vi "Destroy.vi"(0 "reference in":refnum<class "Test Controller.lvclass">, 5 "error in (no error)":errorcluster) -> (14 "reference out":refnum<class "Test Controller.lvclass">, 19 "error out":errorcluster)   [LabVIEW 2016, in "Test Controller.lvclass"]
doc: "Destructor."
uses:
  Test Controller.lvclass
  <vilib>/addons/_AddQ/G#Object/G#Object.lvclass
  C:/Program Files (x86)/National Instruments/LabVIEW 2016/vi.lib/addons/_AddQ/G#Object/G#Object.lvclass
  APP/python_class/python.lvclass
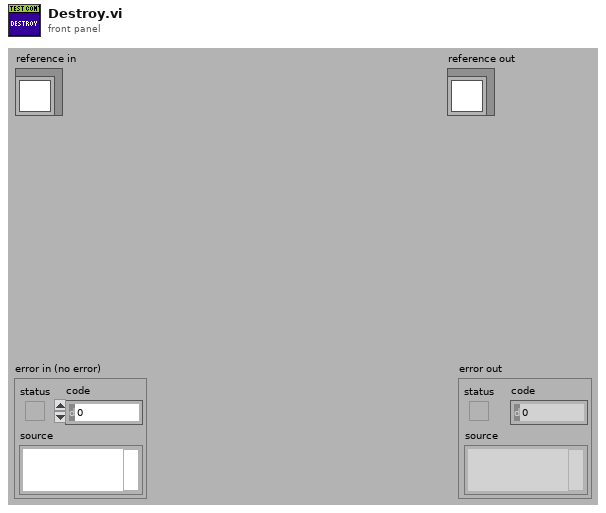
[diagram p1: front panel]
types:
  T1 = typedef "Test Controller.lvclass/ObjectAttributes.ctl" = cluster{"MyAttribute":dbl, "Devices Controller_ref":refnum<class "Devices Controller.lvclass">, "File Controller_ref":refnum<class "File Controller.lvclass">, "Items Controller_ref":refnum<class "Items Controller.lvclass">, "GUI Controller_ref":refnum<class "GUI Controller.lvclass">, "NotificationController_ref":refnum<class "Notification Controller.lvclass">, "PartsTracking Controller_ref":refnum<class "PartsTracking Controller.lvclass">}
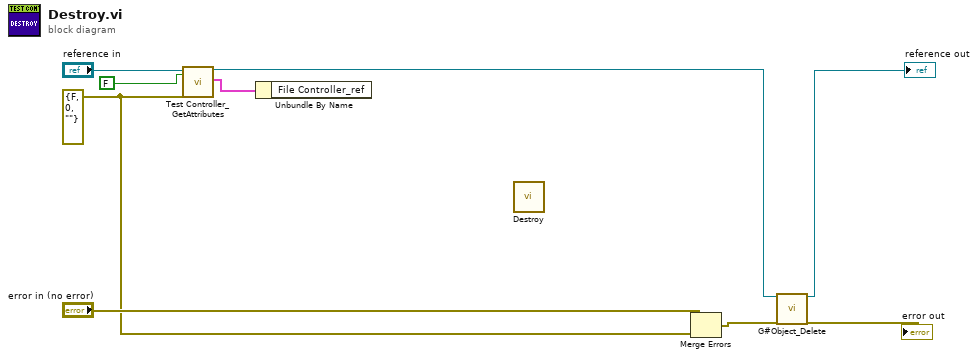
[diagram p0: block diagram]
diagram:
  w10 = errorcluster {"status"=FALSE, "code"=0, "source"=""} ("error in (no error)")
  n1 = call "Test Controller_GetAttributes.vi"("reference in"="reference in", "return data? (T)"=FALSE ("simple info"), "error in (no error)"=w10) -> ("reference out"=w7:refnum<class "Test Controller.lvclass">, "attributes"=w4:T1, "error out"=w2:errorcluster)  [unwired: 13 in, 1 out]
  n2 = Unbundle By Name(w4) -> ("File Controller_ref"=w3:refnum<class "File Controller.lvclass">)
  n3 = call-dynamic "Destroy.vi"() -> ()  [unwired: 18 in, 2 out]
  n4 = Merge Errors("error in (no error)", w10) -> (w9:errorcluster, w1:errorcluster)
  n5 = call <vilib>:"G#Object_Delete.vi"("reference in"=w7, "error in (no error)"=w9) -> ("reference out"=→"reference out":refnum<class "Test Controller.lvclass">, "error out"=→"error out":errorcluster)  [unwired: 16 in]
